vi "Read Measure (Percentage).vi"(8 "error in (no error)":errorcluster, 10 "Node (3)":u8=3 caption="Node" min=3 max=128 step=1, 11 "VISA resource name":refnum<visa-resource-name>) -> (0 "error out":errorcluster, 2 "Measure Percentage":dbl, 3 "VISA resource name out":refnum<visa-resource-name>)   [LabVIEW 2022 SP3, in "Bronkhorst FLOW-BUS.lvlib"]
doc: "Reads the measured value in the instrument. Depending on the type of instrument, the measured value indicates the amount of mass flow or pressure metered by the instrument.\nIn this VI a value between 0-100% will be displayed on the frontpanel, 100% equals capacity and 0% equals 0."
uses:
  Bronkhorst FLOW-BUS.lvlib
  Private/FLOW-BUS RW.ctl
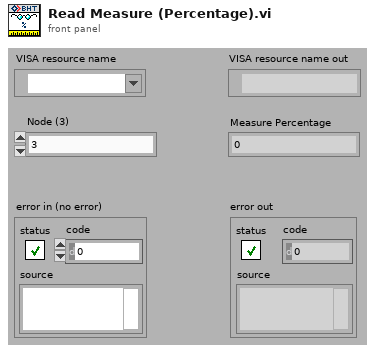
[diagram p1: front panel]
types:
  T1 = typedef "Bronkhorst FLOW-BUS.lvlib/FLOW-BUS RW.ctl" = cluster{"Node Address (3)":u8, "Communication Command":enum16{"Status message", "Send parameter with destination address and 00 response", "Send parameter with destination address", "Request parameter"}, "Process (0)":u16, "Parameter (0)":u16, "Data Type (0: Character)":enum16{"Character", "Integer", "Float or Long", "String"}, "Data for Char or Int (0)":u32, "Data for Float or Long (0)":sgl, "Data for String":string, "Length of Requested String (0)":u8}
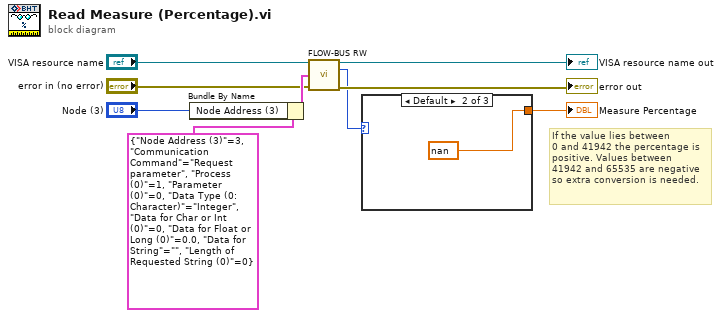
[diagram p0: block diagram]
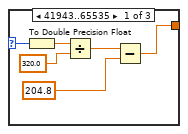
[diagram p2: hidden frame]
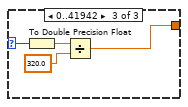
[diagram p3: hidden frame]
diagram:
  # "If the value lies between\n0 and 41942 the percentage is \npositive. Values between \n41942 and 65535 are negative\nso extra conversion is needed."
  n1 = Bundle By Name(cluster=T1 {"Node Address (3)"=3, "Communication Command"=enum."Request parameter", "Process (0)"=1, "Parameter (0)"=0, "Data Type (0: Character)"=enum."Integer", "Data for Char or Int (0)"=0, "Data for Float or Long (0)"=0.0, "Data for String"="", "Length of Requested String (0)"=0} ("FLOW-BUS Command Settings"), "Node Address (3)"="Node (3)") -> (w8:T1)
  n2 = call "FLOW-BUS RW.vi"("VISA resource name"="VISA resource name", "FLOW-BUS Command Settings"=w8, "error in (no error)"="error in (no error)") -> ("VISA resource name out"=→"VISA resource name out":refnum<visa-resource-name>, "Requested Char, Int or Long"=w2:u32, "error out"=→"error out":errorcluster)  [unwired: 8 in, 2 out]
  n3 = case shown="Default" w2 {
    selector: w2 -> [w11 _ w18]
    tunnel: [w14 nan w19] -> w9
    frame 41943..65535 {
      n4 = To Double Precision Float(number=w11) -> (double precision float=w10:dbl)
      n5 = Divide(x=w10, y=320.0) -> (x/y=w12:dbl)
      n6 = Subtract(x=w12, y=204.8) -> (x-y=w14:dbl)
    }
    frame Default {
    }
    frame 0..41942 {
      n7 = To Double Precision Float(number=w18) -> (double precision float=w17:dbl)
      n8 = Divide(x=w17, y=320.0) -> (x/y=w19:dbl)
    }
  }
  "Measure Percentage" <- w9
